vi "KM_Array Select.vi"   [LabVIEW 2015]
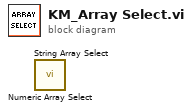
[diagram p0: block diagram]
diagram:
  n1 = call "Numeric Array Select.vi"() -> ()  [unwired: 11 in, 1 out]
  n2 = call "String Array Select.vi"() -> ()  [unwired: 11 in, 1 out]
